vi "trigen.vi"(2 "piezo constant":dbl=1505.255 format="%#_13g", 3 "Invert?":bool=TRUE, 4 "error in":errorcluster, 5 "liczba probek":dbl=10000.0 min=100.0 max=1000000.0 step=10000.0, 6 "scanstart [nm]":dbl(slide)=3000.0 scale=0.0..6000.0, 7 "scansize [nm]":dbl(slide)=1500.0 scale=0.0..5000.0) -> (0 "error out":errorcluster, 1 "Waveform Graph":dbl[](graph))   [LabVIEW 2013]
uses:
  <vilib>/Analysis/NI_AALPro.lvlib
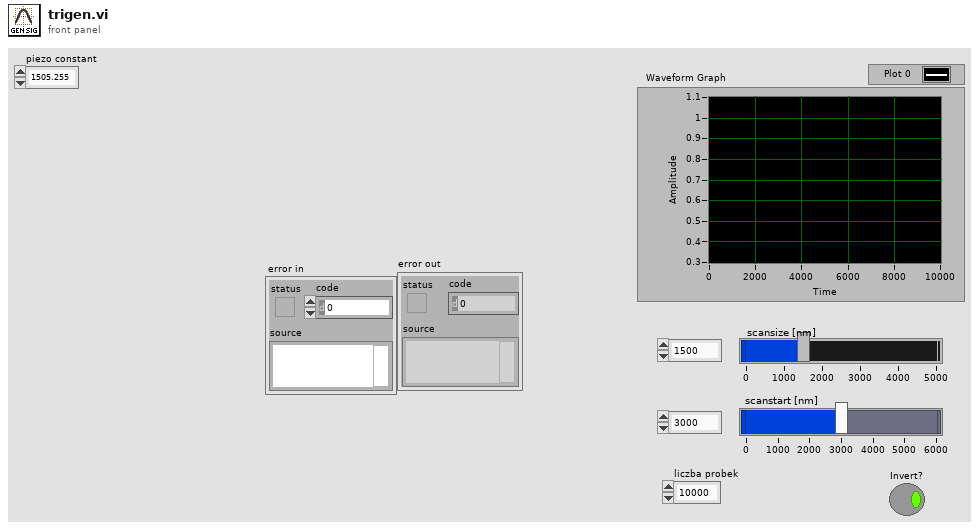
[diagram p1: front panel]
types:
  T1 = enum16{"sine", "cosine", "triangle", "square", "sawtooth", "increasing ramp", "decreasing ramp"}
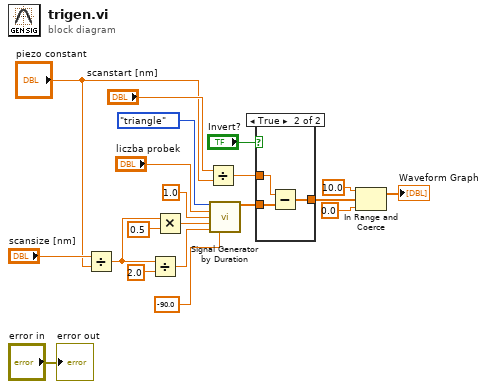
[diagram p0: block diagram]
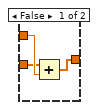
[diagram p2: hidden frame]
diagram:
  n1 = Divide(x="scansize [nm]", y="piezo constant") -> (x/y=w8:dbl)
  n2 = Divide(x=w8, y=2.0) -> (x/y=w13:dbl)
  n3 = Multiply(x=w8, y=0.5) -> (x*y=w11:dbl)
  n4 = Divide(x="scanstart [nm]", y="piezo constant") -> (x/y=w2:dbl)
  n5 = call <vilib>:"Signal Generator by Duration.vi"("signal type"=T1."triangle", "# of samples"="liczba probek", "frequency"=1.0, "amplitude"=w11, "dc offset"=w13, "phase in"=-90.0) -> ("signal"=w12:dbl[])  [unwired: 6 in, 3 out]
  n6 = case shown="True" "Invert?" {
    tunnel: [w21 w25] -> w1
    tunnel: w12 -> [w22 w24]
    tunnel: w2 -> [w23 w26]
    frame False {
      n7 = Add(x=w22, y=w23) -> (x+y=w21:dbl[])
    }
    frame True {
      n8 = Subtract(x=w26, y=w24) -> (x-y=w25:dbl[])
    }
  }
  n9 = In Range and Coerce(upper limit=10.0 ("y"), x=w1, lower limit=0.0 ("y")) -> (coerced(x)=→"Waveform Graph":dbl[])  [unwired: 1 out]
  "error out" <- "error in"
